vi "Save All.vi"(8 "error in (no error)":errorcluster, 11 "StorageService in":refnum<class "StorageService.lvclass">) -> (0 "error out":errorcluster, 3 "StorageService out":refnum<class "StorageService.lvclass">)   [LabVIEW 2014, in "StorageService.lvclass"]
uses:
  StorageService.lvclass
  StorageService.lvclass/StorageService.ctl
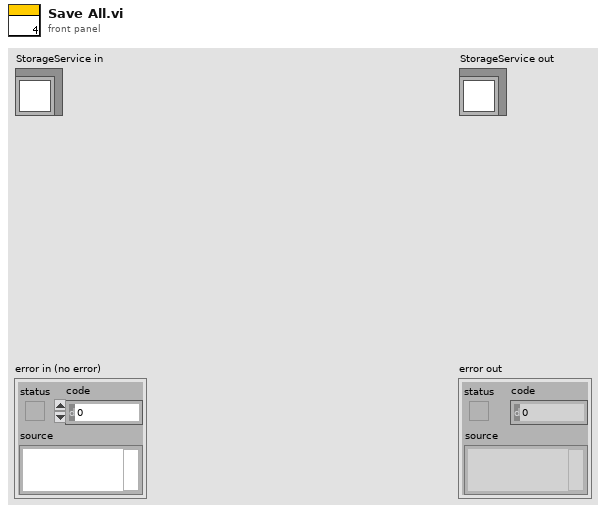
[diagram p1: front panel]
types:
  T1 = typedef "StorageService.lvclass/RegisteredObject.ctl" = cluster{"Name":string, "Is Acquired":bool, "Queue":refnum<queue>, "Message To Send":cluster{"Enqueuer":refnum<class "Message Enqueuer.lvclass">, "Message":refnum<class "ReplayData Msg.lvclass">}, "Save Parameters":variant}
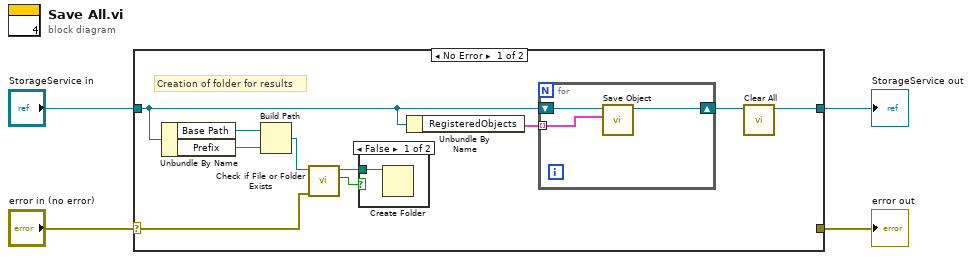
[diagram p0: block diagram]
diagram:
  n1 = case shown="No Error" "error in (no error)" {
    selector: "error in (no error)" -> [w6 w20]
    tunnel: [_ w20] -> w3
    tunnel: [w12 w19] -> w1
    tunnel: "StorageService in" -> [w11 w19]
    frame No Error {
      # "Creation of folder for results"
      n2 = Unbundle By Name(w11) -> ("Base Path"=w10:path, "Prefix"=w9:string)
      n3 = Build Path(base path=w10, name or relative path=w9) -> (appended path=w8:path)
      n4 = call <vilib>:"Check if File or Folder Exists.vi"("error in (no error)"=w6, "path"=w8) -> ("file or folder exists?"=w5:bool, "dup path"=w7:path)  [unwired: 7 in, 1 out]
      n5 = case shown="False" w5 {
        tunnel: w7 -> [w15 _]
        frame False {
          n6 = Create Folder(path (use dialog)=w15) -> ()  [unwired: 2 in, 3 out]
        }
        frame True {
        }
      }
      n7 = Unbundle By Name(w11) -> ("RegisteredObjects"=w14:T1[])
      n8 = for {
        tunnel: w14 -> [w18] mode=indexing
        shift-right: [w16] -> w13
        shift-left: w11 -> [w17]
        n9 = call-dynamic "Save Object.vi"("Object"=w18, "StorageService in"=w17) -> ("StorageService out"=w16:refnum<class "StorageService.lvclass">)  [unwired: 8 in, 1 out]
      }
      n10 = call-dynamic "Clear All.vi"("StorageService in"=w13) -> ("StorageService out"=w12:refnum<class "StorageService.lvclass">)  [unwired: 9 in, 1 out]
    }
    frame Error {
    }
  }
  "error out" <- w3
  "StorageService out" <- w1
